vi "LIN Diag.vi"() -> ()   [LabVIEW 2015]
uses:
  <vilib>/xnet/xnet.llb/XNET Frame LIN.ctl
  <vilib>/xnet/xnet.llb/XNET Frame Type LIN.ctl
  <vilib>/xnet/xnet.llb/XNET Create Session (Frame Input Queued).vi
  <vilib>/xnet/xnet.llb/XNET Create Session (Frame Output Queued).vi
  <vilib>/xnet/xnet.llb/XNET Write (State LIN Schedule Change).vi
  <vilib>/xnet/xnet.llb/XNET Write (Frame LIN).vi
  <vilib>/xnet/xnet.llb/XNET Wait (Transmit Complete).vi
  <vilib>/xnet/xnet.llb/XNET Read (Frame LIN).vi
  <resource>/objmgr/xnet.rc
panel:
  out "error out":errorcluster
  out "data":T1[](array[typedef]) {"event ID" format="%x"; "payload" format="%x"; "timestamp" format="%<%.7X\n%x>T"; "type" items=["LIN Data"=64, "LIN Bus Error"=65, "LIN No Response"=66, "Delay"=224, "Log Trigger"=225, "Start Trigger"=226]; "identifier" format="%x"}
  in  "Frame Payloads to Queue":u8[][](array[numeric]) format="%.0x"
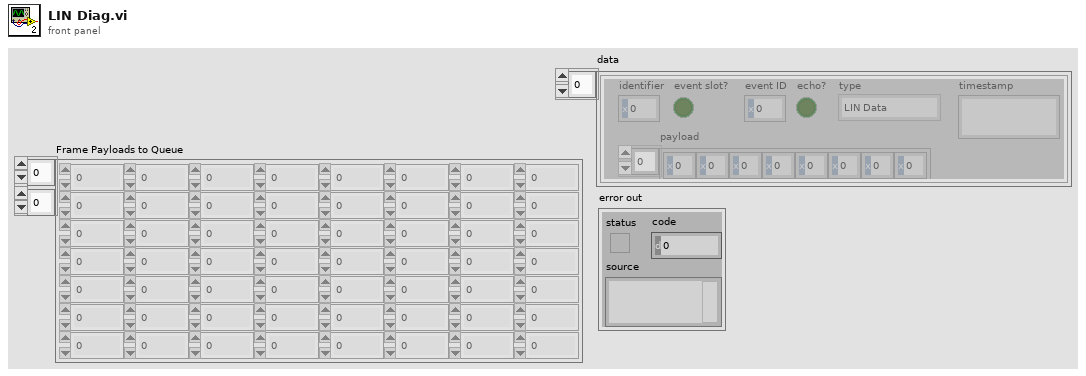
[diagram p1: front panel]
types:
  T1 = typedef "XNET Frame LIN.ctl" = cluster{"timestamp":timestamp, "payload":u8[], "identifier":u32, "type":T2, "event ID":u8, "event slot?":bool, "echo?":bool}
  T2 = typedef "XNET Frame Type LIN.ctl" = u8
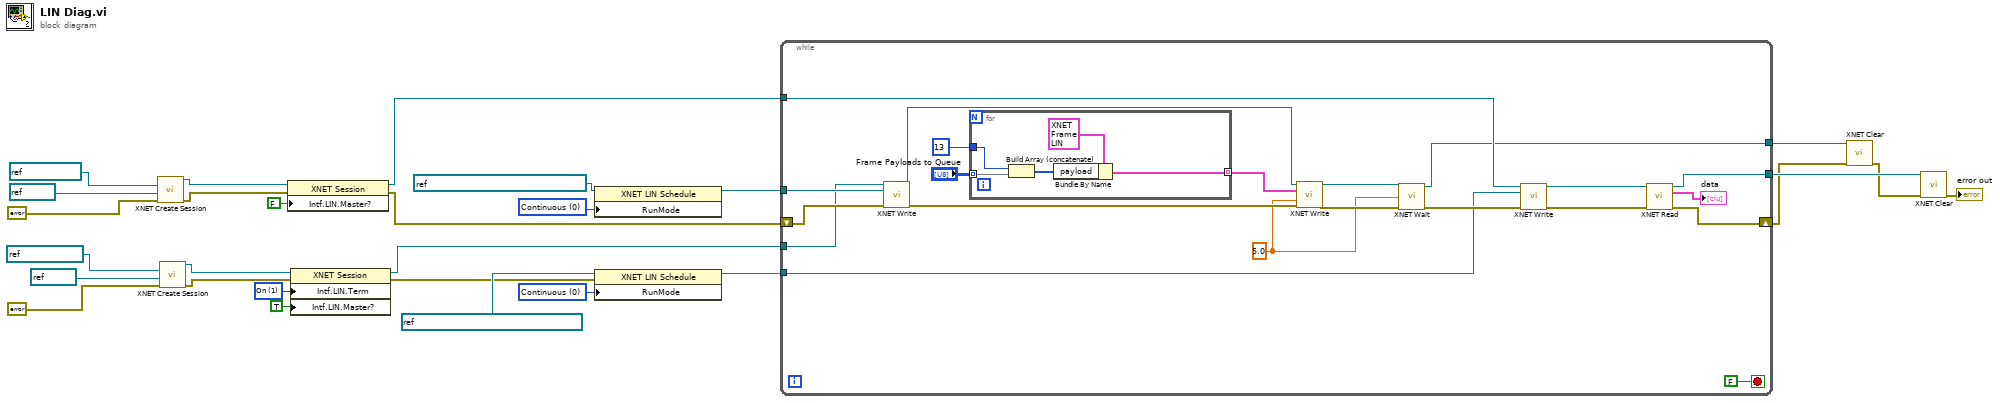
[diagram p0: block diagram]
diagram:
  w20 = u32 0 items=["Continuous", "Once", "Null"] ("Run Mode")
  w21 = u32 0 items=["Continuous", "Once", "Null"] ("Run Mode")
  w25 = u32 1 items=["Off", "On"] ("Interface:LIN:Termination")
  n1 = call-poly <vilib>:"XNET Create Session.vi"("frame"=refnum<k21> "SlaveResp\nCS110501", "interface"=refnum<k21> "LIN2", "error in (no error)"=errorcluster {"status"=FALSE, "code"=0, "source"=""}) -> ("session out"=w28:refnum<k21>, "error out"=w27:errorcluster)  [unwired: 11 in]
  n2 = call-poly <vilib>:"XNET Create Session.vi"("frame"=refnum<k21> "MasterReq\nCS110501", "interface"=refnum<k21> "LIN2", "error in (no error)"=errorcluster {"status"=FALSE, "code"=0, "source"=""}) -> ("session out"=w10:refnum<k21>, "error out"=w26:errorcluster)  [unwired: 11 in]
  n3 = property class="XNET Session"(reference=w28, error in=w27, "Intf.LIN.Master?"=FALSE ("Interface:LIN:Master?")) -> (reference out=w7:refnum<k21>, error out=w11:errorcluster)
  n4 = property class="XNET Session"(reference=w10, error in=w26, "Intf.LIN.Term"=w25, "Intf.LIN.Master?"=TRUE ("Interface:LIN:Master?")) -> (reference out=w9:refnum<k21>, error out=w12:errorcluster)
  n5 = property on="属性节点" class="XNET LIN Schedule"(reference=refnum<k21> "CEMLIN3DiagRequestSchedule\nCS110501" ("XNET LIN Schedule"), "RunMode"=w21) -> (reference out=w13:refnum<k21>)  [unwired: 1 in, 1 out]
  n6 = property on="属性节点" class="XNET LIN Schedule"(reference=refnum<k21> "CEMLIN3DiagResponseSchedule\nCS110501" ("XNET LIN Schedule"), error in=w12, "RunMode"=w20) -> (reference out=w6:refnum<k21>)  [unwired: 1 out]
  n7 = while {
    tunnel: w13 -> [w49]
    shift-right: [w35] -> w2
    shift-left: w11 -> [w36]
    tunnel: w9 -> [w34]
    tunnel: w7 -> [w33]
    tunnel: w6 -> [w32]
    tunnel: [w31] -> w5
    tunnel: [w30] -> w4
    stop <- FALSE stop-if-true
    w41 = 5.0 ("timeout (10)")
    n8 = call-poly <vilib>:"XNET Write.vi"("session in"=w34, "data"=w49, "error in (no error)"=w36) -> ("session out"=w46:refnum<k21>, "error out"=w44:errorcluster)  [unwired: 11 in]
    n9 = for {
      tunnel: u8 13 ("identifier") -> [w54]
      tunnel: "Frame Payloads to Queue" -> [w53] mode=indexing
      tunnel: [w51] -> w45 mode=indexing
      n10 = Build Array (concatenate)(w54, w53) -> (w50:u8[])
      n11 = Bundle By Name(cluster=T1 {"timestamp"=timestamp(0 s since 1904-01-01), "payload"=[], "identifier"=0, "type"=64, "event ID"=0, "event slot?"=FALSE, "echo?"=FALSE} ("LIN frame"), "payload"=w50) -> (w51:T1)
    }
    n12 = call-poly <vilib>:"XNET Write.vi"("session in"=w46, "data"=w45, "timeout (10)"=w41, "error in (no error)"=w44) -> ("session out"=w42:refnum<k21>, "error out"=w43:errorcluster)  [unwired: 10 in]
    n13 = call-poly <vilib>:"XNET Wait.vi"("session in"=w42, "timeout (10)"=w41, "error in (no error)"=w43) -> ("session out"=w31:refnum<k21>, "error out"=w40:errorcluster)  [unwired: 11 in]
    n14 = call-poly <vilib>:"XNET Write.vi"("session in"=w33, "data"=w32, "error in (no error)"=w40) -> ("session out"=w39:refnum<k21>, "error out"=w38:errorcluster)  [unwired: 11 in]
    n15 = call-poly <vilib>:"XNET Read.vi"("session in"=w39, "error in (no error)"=w38) -> ("session out"=w30:refnum<k21>, "data"=→"data":T1[], "error out"=w35:errorcluster)  [unwired: 10 in, 1 out]
  }
  n16 = call <vilib>:"XNET Clear.vi"("session in"=w5, "error in (no error)"=w2) -> ("error out"=w3:errorcluster)  [unwired: 13 in]
  n17 = call <vilib>:"XNET Clear.vi"("session in"=w4, "error in (no error)"=w3) -> ("error out"=→"error out":errorcluster)  [unwired: 13 in]
